vi "Read ref.vi"(8 "error in (no error)":errorcluster, 11 "SqlMapper in":refnum<class "DapperMapper.lvclass">) -> (0 "error out":errorcluster, 2 "SQLMapper ref":T1, 3 "SqlMapper out":refnum<class "DapperMapper.lvclass">)   [LabVIEW 2020, in "ORM_Dapper.lvlib" / "DapperMapper.lvclass"]
uses:
  DapperMapper.lvclass
  dapper_sqlmapper_ref.ctl
  C:/Viviota/Projects/R&D/LabVIEW_ORM/source/src/libraries/dapper/Dapper.dll
  libraries/dapper/Dapper.dll
  ORM_Dapper.lvlib
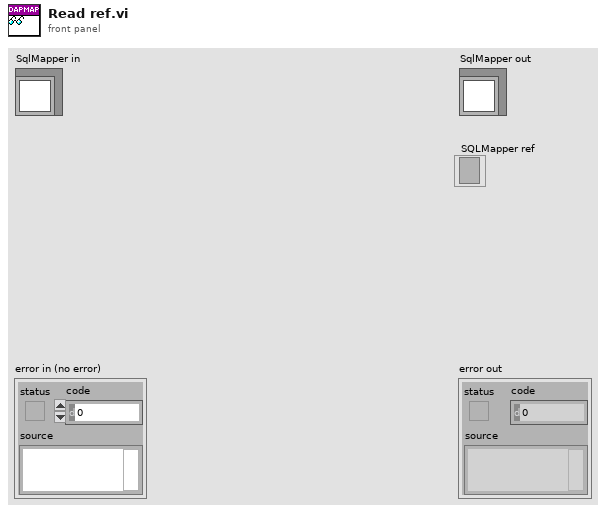
[diagram p1: front panel]
types:
  T1 = typedef "ORM_Dapper.lvlib/dapper_sqlmapper_ref.ctl" = refnum<k24>
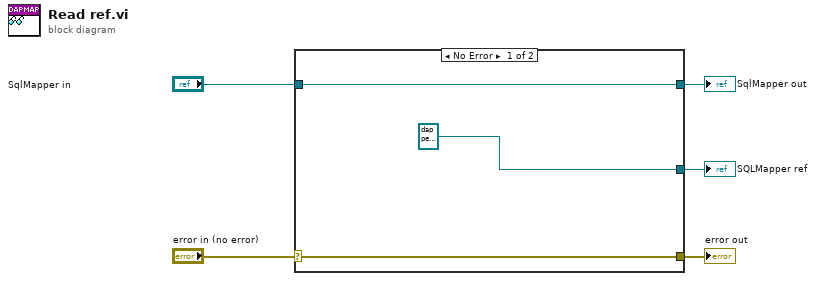
[diagram p0: block diagram]
diagram:
  n1 = case shown="No Error" "error in (no error)" {
    selector: "error in (no error)" -> [w8 w9]
    tunnel: [w8 w9] -> w4
    tunnel: [w7 w10] -> w2
    tunnel: "SqlMapper in" -> [w7 w10]
    tunnel: [T1 refnum ("ref") _] -> w1
    frame No Error {
    }
    frame Error {
    }
  }
  "error out" <- w4
  "SqlMapper out" <- w2
  "SQLMapper ref" <- w1
